vi "N5232-PNA_AvgDone.vi"(0 "Session In":refnum<visa-resource-name>="TCPIP0::169.254.70.180::inst0::INSTR", 5 "input":i32=1, 11 "error in":errorcluster {"code" format="%.0x"}) -> (3 "Avg_Done?(t)":bool, 4 "Session Out":refnum<visa-resource-name>, 15 "error out":errorcluster {"code" format="%.0x"})   [LabVIEW 2018]
doc: "Launches the Instrument I/O Assistant, which you can use to communicate with message-based instruments and graphically parse the response. For example you can communicate with an instrument that uses a serial, Ethernet, or GPIB interface."
uses:
  Keysight PNA Series/Keysight PNA Series.lvlib
panel:
  out "Error Message":string
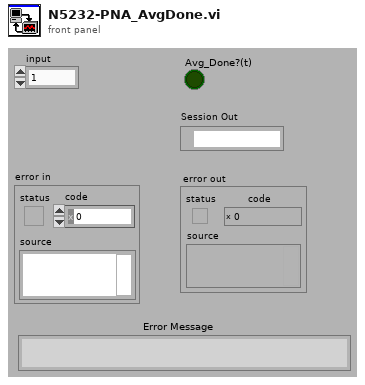
[diagram p1: front panel]
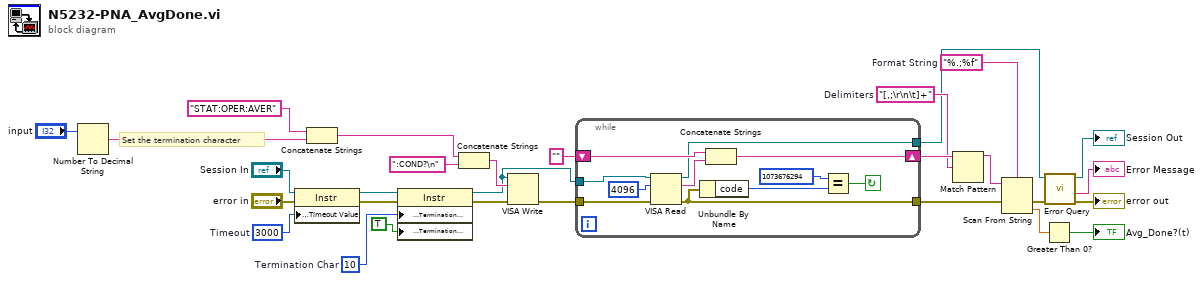
[diagram p0: block diagram]
diagram:
  w9 = "[,;\r\n\t]+"  # Delimiters
  w10 = "%.;%f"  # Format String
  w23 = u8 10  # Termination Char
  w27 = u32 3000  # Timeout
  # "Set the termination character"
  n1 = Number To Decimal String(number="input") -> (decimal integer string=w20:string)  [unwired: 1 out]
  n2 = property class="Instr"(reference="Session In", error in="error in", "General Settings:Timeout Value"=w27) -> (reference out=w22:refnum<visa-resource-name>, error out=w25:errorcluster)
  n3 = Concatenate Strings("STAT:OPER:AVER" ("staticText"), w20) -> (w16:string)
  n4 = property class="Instr"(reference=w22, error in=w25, "Message Based Settings:Termination Character"=w23, "Message Based Settings:Termination Character Enable"=TRUE ("enable")) -> (reference out=w8:refnum<visa-resource-name>, error out=w24:errorcluster)
  n5 = Concatenate Strings(w16, ":COND?\n" ("StaticText")) -> (w17:string)
  n6 = VISA Write(VISA resource name=w8, write buffer=w17, error in (no error)=w24) -> (error out=w18:errorcluster)  [unwired: 2 out]
  n7 = while {
    tunnel: w8 -> [w31]
    shift-left: "" -> [w34]
    shift-right: [w33] -> w12
    tunnel: w18 -> [w32]
    tunnel: [w36] -> w13
    tunnel: [w30] -> w4
    stop <- w38 continue-if-true
    n8 = VISA Read(VISA resource name=w31, byte count=u32 4096 ("byte count (0)"), error in (no error)=w32) -> (VISA resource name out=w30:refnum<visa-resource-name>, read buffer=w35:string, error out=w36:errorcluster)  [unwired: 1 out]
    n9 = Unbundle By Name(w36) -> ("code"=w39:i32)
    n10 = Concatenate Strings(w34, w35) -> (w33:string)
    n11 = Equal?(x=1073676294, y=w39) -> (x = y?=w38:bool)
  }
  n12 = Match Pattern(string=w12, regular expression=w9) -> (before substring=w11:string)  [unwired: 1 in, 3 out]
  n13 = Scan From String(format string=w10, input string=w11, error in=w13) -> (error out=w5:errorcluster, output 1=w7:dbl)  [unwired: 2 in, 2 out]
  n14 = Greater Than 0?(x=w7) -> (x > 0?=→"Avg_Done?(t)":bool)
  n15 = call "Error Query.vi"("error in (no error)"=w5, "VISA resource name"=w4) -> ("error out"=→"error out":errorcluster, "Error Message"=→"Error Message":string, "VISA resource name out"=→"Session Out":refnum<visa-resource-name>)  [unwired: 6 in, 1 out]
